vi "test_all_riccati.vi"(8 "error in (no error)":errorcluster) -> (0 "error out":errorcluster, 3 "All Tests Passed":bool)   [LabVIEW 2019]
panel:
  out "Test 4N":bool
  out "Test 3N":bool
  out "Test 2N":bool
  out "Test 1N":bool
  out "Test 5":bool
  out "Test 4":bool
  out "Test 3":bool
  out "Test 2":bool
  out "Test 1":bool
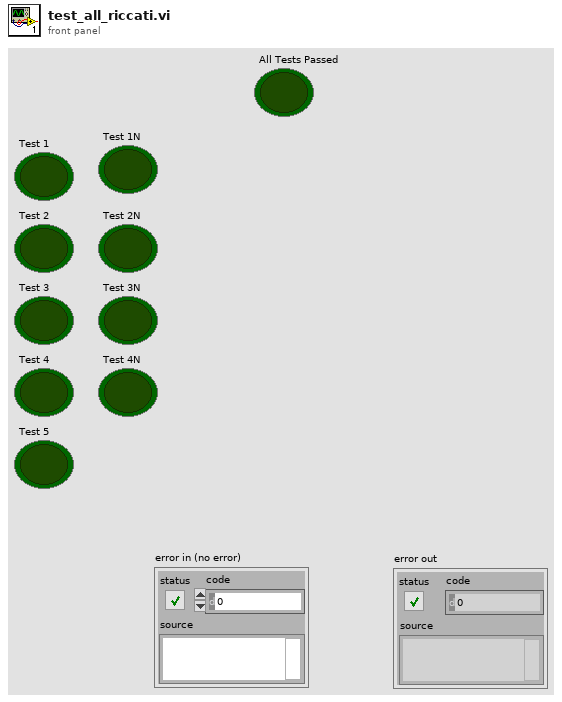
[diagram p1: front panel]
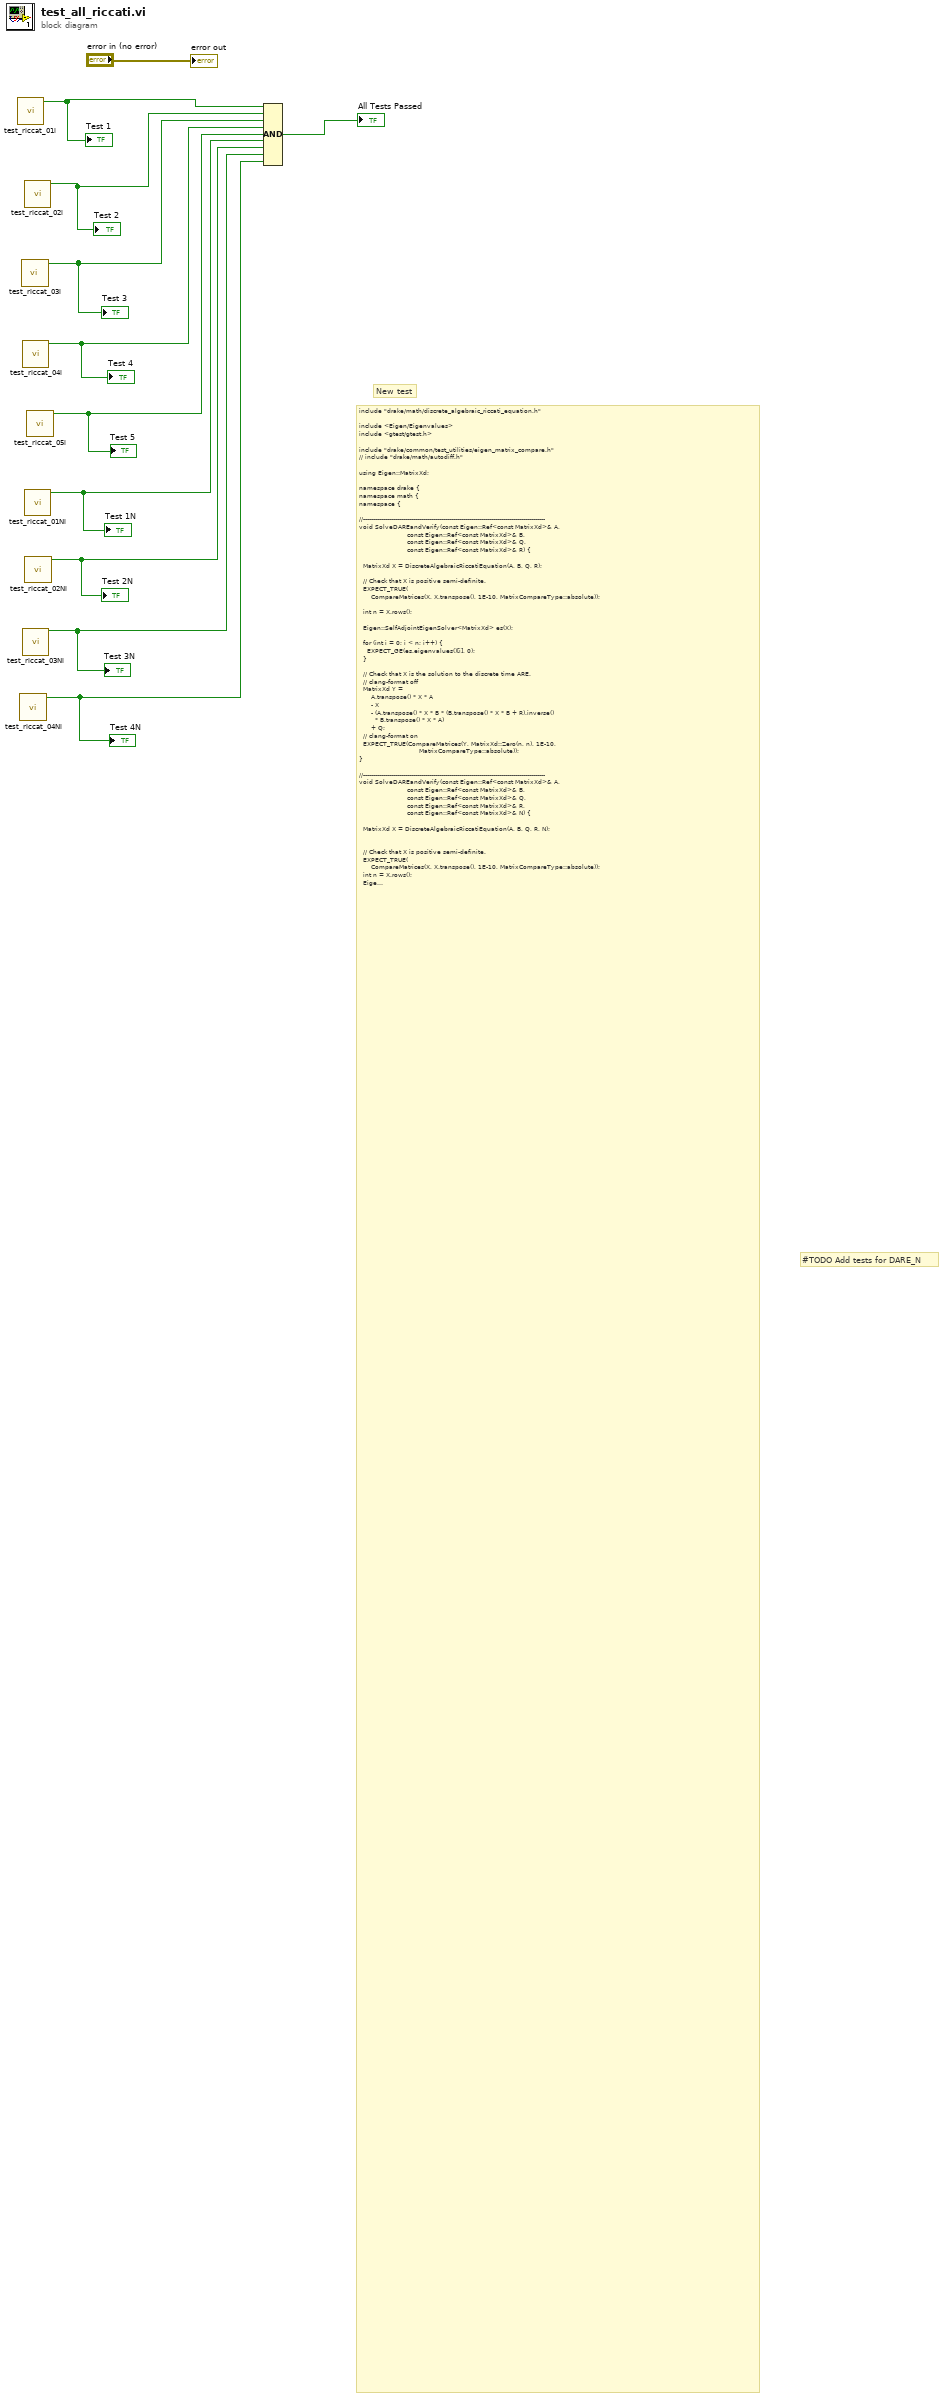
[diagram p0: block diagram]
diagram:
  # "#TODO Add tests for DARE_N"
  # "New test"
  # "include \"drake/math/discrete_algebraic_riccati_equation.h\"\n\ninclude <Eigen/Eigenvalues>\ninclude <gtest/gtest.h>\n\ninclude \"drake/common/test_utilities/eigen_matrix_compare.h\"\n// include \"drake/math/autodiff.h\"\n\nusing Eigen::MatrixXd;\n\nnamespace drake {\nnamespace math {\nnamespace {\n\n//-------------------------------------------------------------------------------------------\nvoid SolveDAREandVerify(const Eigen::Ref<const MatrixXd>& A,\n                        const Eigen::Ref<const MatrixXd>& B,\n                        const Eigen::Ref<const MatrixXd>& Q,\n                        const Eigen::Ref<const MatrixXd>& R) {\n\n  MatrixXd X = DiscreteAlgebraicRiccatiEquation(A, B, Q, R);\n\n  // Check that X is positive semi-definite.\n  EXPECT_TRUE(\n      CompareMatrices(X, X.transpose(), 1E-10, MatrixCompareType::absolute));\n\n  int n = X.rows();\n\n  Eigen::SelfAdjointEigenSolver<MatrixXd> es(X);\n\n  for (int i = 0; i < n; i++) {\n    EXPECT_GE(es.eigenvalues()[i], 0);\n  }\n\n  // Check that X is the solution to the discrete time ARE.\n  // clang-format off\n  MatrixXd Y =\n      A.transpose() * X * A\n      - X\n      - (A.transpose() * X * B * (B.transpose() * X * B + R).inverse()\n        * B.transpose() * X * A)\n      + Q;\n  // clang-format on\n  EXPECT_TRUE(CompareMatrices(Y, MatrixXd::Zero(n, n), 1E-10,\n                              MatrixCompareType::absolute));\n}\n\n//-------------------------------------------------------------------------------------------\nvoid SolveDAREandVerify(const Eigen::Ref<const MatrixXd>& A,\n                        const Eigen::Ref<const MatrixXd>& B,\n                        const Eigen::Ref<const MatrixXd>& Q,\n                        const Eigen::Ref<const MatrixXd>& R,\n                        const Eigen::Ref<const MatrixXd>& N) {\n\n  MatrixXd X = DiscreteAlgebraicRiccatiEquation(A, B, Q, R, N);\n\n\n  // Check that X is positive semi-definite.\n  EXPECT_TRUE(\n      CompareMatrices(X, X.transpose(), 1E-10, MatrixCompareType::absolute));\n  int n = X.rows();\n  Eigen::SelfAdjointEigenSolver<MatrixXd> es(X);\n  for (int i = 0; i < n; i++) {\n    EXPECT_GE(es.eigenvalues()[i], 0);\n  }\n  // Check that X is the solution to the discrete time ARE.\n  // clang-format off\n  MatrixXd Y =\n      A.transpose() * X * A\n      - X\n      - ((A.transpose() * X * B + N) * (B.transpose() * X * B + R).inverse()\n        * (B.transpose() * X * A + N.transpose()))\n      + Q;\n  // clang-format on\n  EXPECT_TRUE(CompareMatrices(Y, MatrixXd::Zero(n, n), 1E-10,\n                              MatrixCompareType::absolute));\n}\n\n//-------------------------------------------------------------------------------------------\nGTEST_TEST(DARE, SolveDAREandVerify) {\n\n//-------------------------------------------------------------------------------------------\n  // Test 1: non-invertible A\n  // Example 2 of \"On the Numerical Solution of the Discrete-Time Algebraic\n  // Riccati Equation\"\n  int n1 = 4, m1 = 1;\n  MatrixXd A1(n1, n1), B1(n1, m1), Q1(n1, n1), R1(m1, m1);\n  A1 << 0.5, 1, 0, 0, 0, 0, 1, 0, 0, 0, 0, 1, 0, 0, 0, 0;\n  B1 << 0, 0, 0, 1;\n  Q1 << 1, 0, 0, 0, 0, 0, 0, 0, 0, 0, 0, 0, 0, 0, 0, 0;\n  R1 << 0.25;\n  SolveDAREandVerify(A1, B1, Q1, R1);\n\n  MatrixXd Aref1(n1, n1);\n  Aref1 << 0.25, 1, 0, 0, 0, 0, 1, 0, 0, 0, 0, 1, 0, 0, 0, 0;\n  SolveDAREandVerify(   A1, \n                                          B1, \n                                          ( A1 - Aref1).transpose() * Q1 * (A1 - Aref1),\n                                          B1.transpose() * Q1 * B1 + R1, \n                                         (A1 - Aref1).transpose() * Q1 * B1);\n\n//-------------------------------------------------------------------------------------------\n  // Test 2: invertible A\n  int n2 = 2, m2 = 1;\n  MatrixXd A2(n2, n2), B2(n2, m2), Q2(n2, n2), R2(m2, m2);\n  A2 << 1, 1, 0, 1;\n  B2 << 0, 1;\n  Q2 << 1, 0, 0, 0;\n  R2 << 0.3;\n  SolveDAREandVerify(A2, B2, Q2, R2);\n\n  MatrixXd Aref2(n2, n2);\n  Aref2 << 0.5, 1, 0, 1;\n  SolveDAREandVerify(    A2, \n                                           B2,\n                                          (A2 - Aref2).transpose() * Q2 * (A2 - Aref2),\n                                          B2.transpose() * Q2 * B2 + R2, \n                                          (A2 - Aref2).transpose() * Q2 * B2);\n\n//-------------------------------------------------------------------------------------------\n  // Test 3: the first generalized eigenvalue of (S,T) is stable\n  int n3 = 2, m3 = 1;\n  MatrixXd A3(n3, n3), B3(n3, m3), Q3(n3, n3), R3(m3, m3);\n  A3 << 0, 1, 0, 0;\n  B3 << 0, 1;\n  Q3 << 1, 0, 0, 1;\n  R3 << 1;\n  SolveDAREandVerify(A3, B3, Q3, R3);\n\n  MatrixXd Aref3(n3, n3);\n  Aref3 << 0, 0.5, 0, 0;\n  SolveDAREandVerify(   A3, \n                                          B3,  \n                                          (A3 - Aref3).transpose() * Q3 * (A3 - Aref3),\n                                          B3.transpose() * Q3 * B3 + R3, \n                                         (A3 - Aref3).transpose() * Q3 * B3);\n\n//-------------------------------------------------------------------------------------------\n  // Test 4: A = B = Q = R = I_2 (2-by-2 identity matrix)\n  const Eigen::MatrixXd A4{Eigen::Matrix2d::Identity()};\n  const Eigen::MatrixXd B4{Eigen::Matrix2d::Identity()};\n  const Eigen::MatrixXd Q4{Eigen::Matrix2d::Identity()};\n  const Eigen::MatrixXd R4{Eigen::Matrix2d::Identity()};\n\n  SolveDAREandVerify(A4, B4, Q4, R4);\n\n  const Eigen::MatrixXd N4{Eigen::Matrix2d::Identity()};\n\n  SolveDAREandVerify(A4, B4, Q4, R4, N4);\n}\n}  // namespace\n}  // namespace math\n}  // namespace drake"
  n1 = call "test_riccat_01i.vi"() -> ("All Tests Passed"=w10:bool)  [unwired: 11 in]
  "Test 1" <- w10
  n2 = call "test_riccat_04Ni.vi"() -> ("All Tests Passed"=w1:bool)  [unwired: 11 in]
  "Test 4N" <- w1
  n3 = call "test_riccat_03i.vi"() -> ("All Tests Passed"=w8:bool)  [unwired: 11 in]
  "Test 3" <- w8
  n4 = call "test_riccat_04i.vi"() -> ("All Tests Passed"=w7:bool)  [unwired: 11 in]
  "Test 4" <- w7
  n5 = call "test_riccat_03Ni.vi"() -> ("All Tests Passed"=w2:bool)  [unwired: 11 in]
  "Test 3N" <- w2
  n6 = call "test_riccat_02i.vi"() -> ("All Tests Passed"=w9:bool)  [unwired: 11 in]
  "Test 2" <- w9
  n7 = call "test_riccat_01Ni.vi"() -> ("All Tests Passed"=w3:bool)  [unwired: 11 in]
  "Test 1N" <- w3
  n8 = call "test_riccat_02Ni.vi"() -> ("All Tests Passed"=w4:bool)  [unwired: 11 in]
  "Test 2N" <- w4
  n9 = call "test_riccat_05i.vi"() -> ("All Tests Passed"=w6:bool)  [unwired: 11 in]
  "Test 5" <- w6
  n10 = Compound Arithmetic op=AND(w10, w9, w8, w7, w6, w3, w4, w2, w1) -> (→"All Tests Passed":bool)
  "error out" <- "error in (no error)"
